vi "global variable-賭金回傳.vi"() -> ()   [LabVIEW 2014]
panel:
  out "賭金回傳":i32
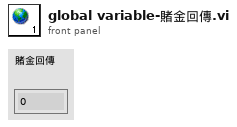
[diagram p1: front panel]
diagram:
